vi "Durchflussanpassung.vi"(8 "Offset":sgl, 9 "Endpunkt":sgl, 11 "Eingang":sgl) -> (3 "Ausgang":dbl)   [LabVIEW 2020, in "Allgemein.lvlib"]
uses:
  Allgemein.lvlib
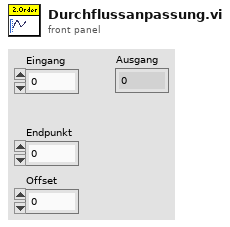
[diagram p1: front panel]
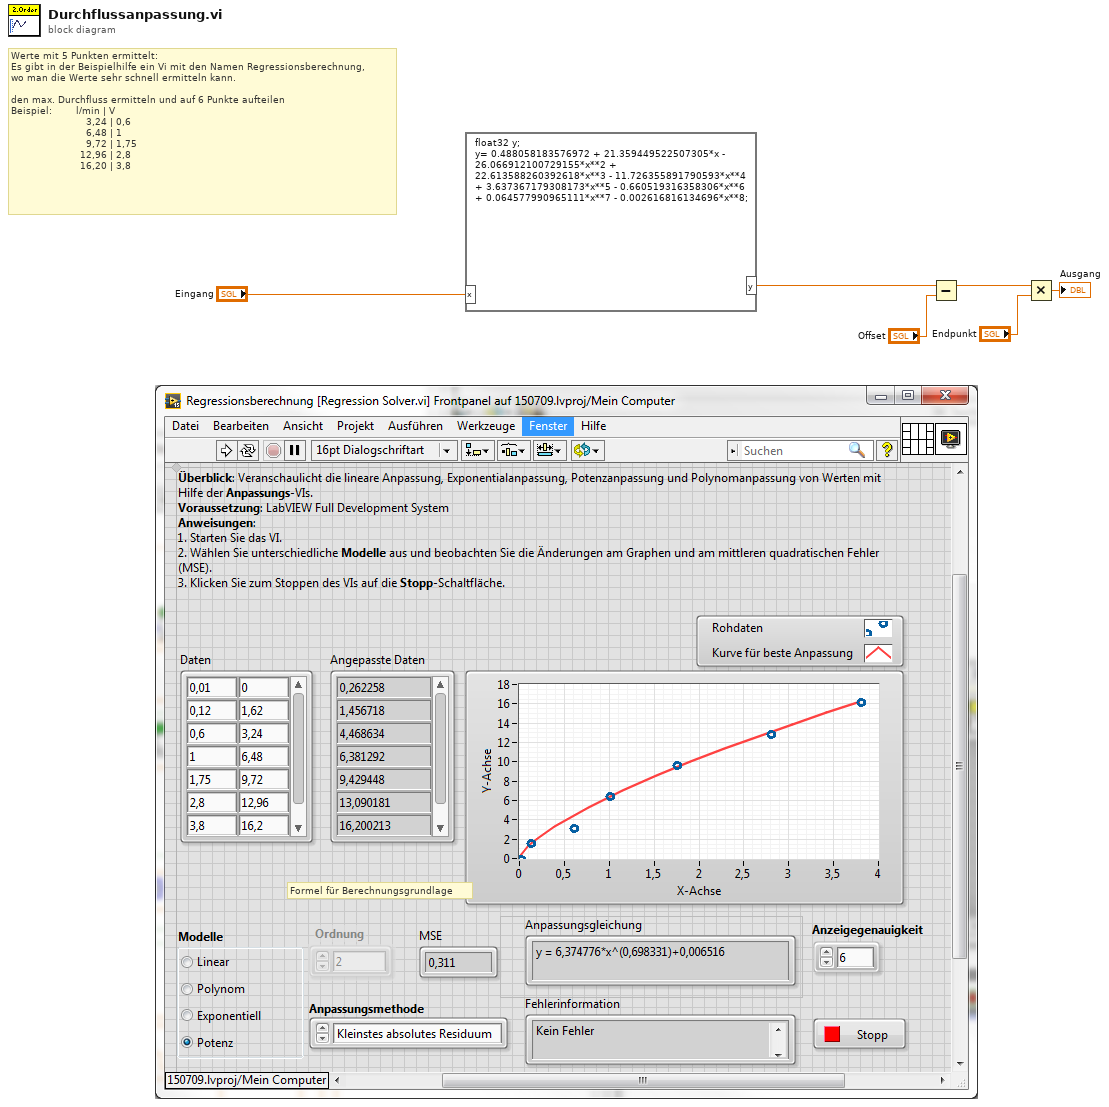
[diagram p0: block diagram]
diagram:
  # "Formel für Berechnungsgrundlage"
  # "Werte mit 5 Punkten ermittelt:\nEs gibt in der Beispielhilfe ein Vi mit den Namen Regressionsberechnung,\nwo man die Werte sehr schnell ermitteln kann.\n\nden max. Durchfluss ermitteln und auf 6 Punkte aufteilen\nBeispiel:        l/min | V\n                         3,24 | 0,6\n                         6,48 | 1\n                         9,72 | 1,75\n                       12,96 | 2,8\n                       16,20 | 3,8"
  n1 = formula code="float32 y;\ny= 0.488058183576972 + 21.359449522507305*x - 26.066912100729155*x**2 + 22.613588260392618*x**3 - 11.726355891790593*x**4 + 3.637367179308173*x**5 - 0.660519316358306*x**6 + 0.064577990965111*x**7 - 0.002616816134696*x**8;"("x"="Eingang") -> ("y"=w1:sgl)
  n2 = Subtract(x=w1, y="Offset") -> (x-y=w4:sgl)
  n3 = Multiply(x=w4, y="Endpunkt") -> (x*y=→"Ausgang":sgl)
